vi "Launcher.vi"() -> ()   [LabVIEW 2012]
uses:
  State_Machine_Enum.ctl
  RefnameEnum.ctl
  Sally_Dashboard_2014/DBNameEnum.ctl
  Robot Global Data.vi
  <vilib>/addons/control/pid/pid.llb/PID (DBL).vi
  <vilib>/addons/control/pid/NI_PID_pid.lvlib
panel:
  out "Analog Signal":dbl(graph)
  in  "ControllerMultiplier":dbl=3000.0
  out "rpm":dbl
  out "motor output":dbl
  out "Time Chart":dbl(graph)
  out "Time Difference":dbl
  in  "Rate (unit/s)":dbl=10.0
  out "State":T1
  out "Value":dbl
  out "Stopped":bool
  out "MotorInput Chart":dbl(graph)=1.0
  out "RPM Chart":dbl(graph)=2105.9590349511814
  out "LauncherTargetRPM":dbl
  in  "PID gains":T2={"proportional gain (Kc)"=0.002, "integral time (Ti, min)"=0.005, "derivative time (Td, min)"=0.0} {"derivative time (Td, min)" step=0.0001 format="%.6f"; "integral time (Ti, min)" step=0.0001 format="%.6f"; "proportional gain (Kc)" step=0.0001 format="%.6f"}
  in  "output range":cluster{"output high":dbl, "output low":dbl}={"output high"=1.0, "output low"=0.0} {"output low" step=0.1 format="%.2f"; "output high" step=0.1 format="%.2f"}
  # "NOTE: UseEncoder\nmust be true in order\nto run PID"
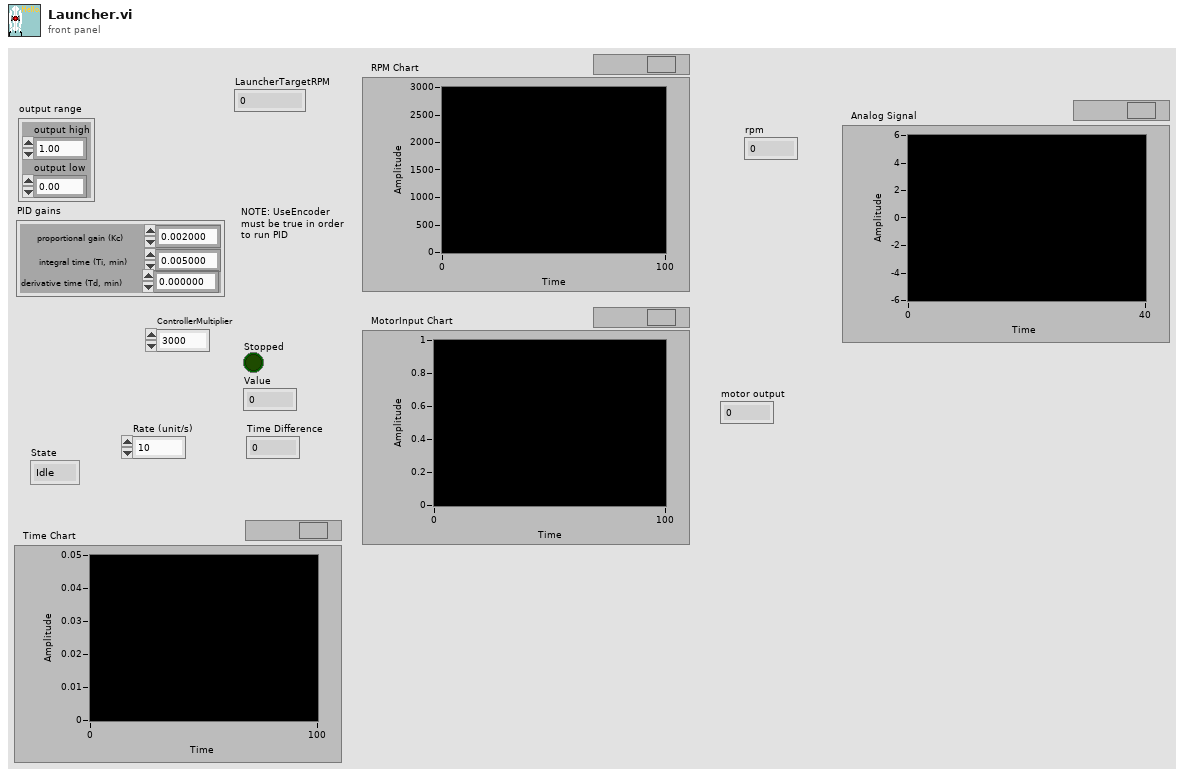
[diagram p1: front panel]
types:
  T1 = typedef "State_Machine_Enum.ctl" = enum16{"Idle", "Start", "Do", "Stop", "Init"}
  T2 = cluster{"proportional gain (Kc)":dbl, "integral time (Ti, min)":dbl, "derivative time (Td, min)":dbl}
  T3 = typedef "RefnameEnum.ctl" = enum16{"FireLauncher", "Climber", "Shield", "TankDrive", "DriveEncoderL", "DriveEncoderR", "LauncherMotorRPM", "LauncherEncoderAnalog", "LauncherEncoderRPM", "ShooterLS", "DriveAlignLSLeft", "DriveAlignLSRight", "ClimbingLS", "LauncherEncoderAngle", "LauncherMotorAngle", "Gamepad1", "Gamepad2", "Compressor", "ClimbWeightSol3", "ClimbWeightSol4"}
  T4 = typedef "DBNameEnum.ctl" = enum16{"AutoInstructions", "DriveLoopTime", "DriveAlignLSLeft", "DriveAlignLSRight", "Use2DriveAlign", "ClimbLS", "LauncherAngleMatches", "FrameworkVersion", "sLauncherAngle", "LauncherTargetAngle", "sLauncherRPM", "LauncherTargetRPM", "sDriveDistance", "LauncherMotorValue", "PullbackTol", "FireTol", "LauncherRPMTol", "LauncherAngleTol", "InitialWait", "WaitBetweenLaunch", "AnglePresets", "RPMPresets", "UseAngleEncoder", "UseLauncherEncoder", "UseLauncherPID", "QSWaitBeforeFire", "QSWaitBeforeRetract", "AngleForwardValue", "AngleBackwardValue", "UseClusterArray", "BackupAuto", "ReverseDriveIndicate", "HalfSpeedFactor"}
  T5 = typedef "LoopDisable.ctl" = cluster{"Climb.vi":bool, "LauncherAngle.vi":bool, "Launcher.vi":bool, "ArmControl.vi":bool, "WinchMotor.vi":bool, "ReadDriveEncoder.vi":bool}
  T6 = typedef "WPI_CounterDevRef.ctl" = cluster{"DevStatus":errorcluster, "CntIndex":T7}
  T7 = typedef "FPGA_CounterCtrSystemIndex.ctl" = enum8{"Ctr 0", "Ctr 1", "Ctr 2", "Ctr 3", "Ctr 4", "Ctr 5", "Ctr 6", "Ctr 7", "Invalid"}
  T8 = typedef "WPI_EncoderDevRef.ctl" = cluster{"DevStatus":errorcluster, "EncoderIndex":T9, "CounterIndex":T7, "DistancePerCount":dbl, "Decoding Type":T10}
  T9 = typedef "FPGA_EncoderIdx.ctl" = enum8{"Enc 0", "Enc 1", "Enc 2", "Enc 3", "Invalid"}
  T10 = typedef "WPI_EncoderType.ctl" = enum16{"1x", "2x", "4x"}
  T11 = typedef "WPI_AnalogChannelDevRef.ctl" = cluster{"DevStatus":errorcluster, "Analog Module":T12, "Analog Channel":T13}
  T12 = typedef "FPGA_TypedefAnalogModule.ctl" = enum16{"Analog Module 1", "Analog Module 2"}
  T13 = typedef "FPGA_AIChannel.ctl" = enum8{"AI 1", "AI 2", "AI 3", "AI 4", "AI 5", "AI 6", "AI 7", "AI 8", "Invalid"}
  T14 = typedef "WPI_MotorControlDeviceRef.ctl" = cluster{"DeviceStatus":errorcluster, "Type":enum16{"PWM", "CAN"}, "PWM":cluster{"Digital Module":T15, "PWM Channel":T16, "DeadBand":T17}, "CAN":cluster{"Device Number":u8, "Control Mode":T18, "Semaphore":T19, "Max Vout":dbl}, "Invert":bool, "TransformRef":T20, "InvTransformRef":T20}
  T15 = typedef "FPGA_TypedefDigitalModule.ctl" = enum16{"Digital Module 1", "Digital Module 2"}
  T16 = typedef "FPGA_DIOPWMChannel.ctl" = enum8{"PWM 1", "PWM 2", "PWM 3", "PWM 4", "PWM 5", "PWM 6", "PWM 7", "PWM 8", "PWM 9", "PWM 10", "Invalid"}
  T17 = typedef "WPI_PWMDeadband.ctl" = cluster{"Name":string, "maxPositivePwm":i32, "minPositivePwm":i32, "centerPwm":i32, "maxNegativePwm":i32, "minNegativePwm":i32, "angularRange":u16}
  T18 = typedef "WPI_CANJaguar_ControlMode.ctl" = enum8{"Percent VBus", "Current", "Speed", "Position", "Voltage"}
  T19 = typedef "Semaphore RefNum" = refnum<k1>
  T20 = typedef "WPI_PWMTransform_ConPane.ctl" = refnum<vi>
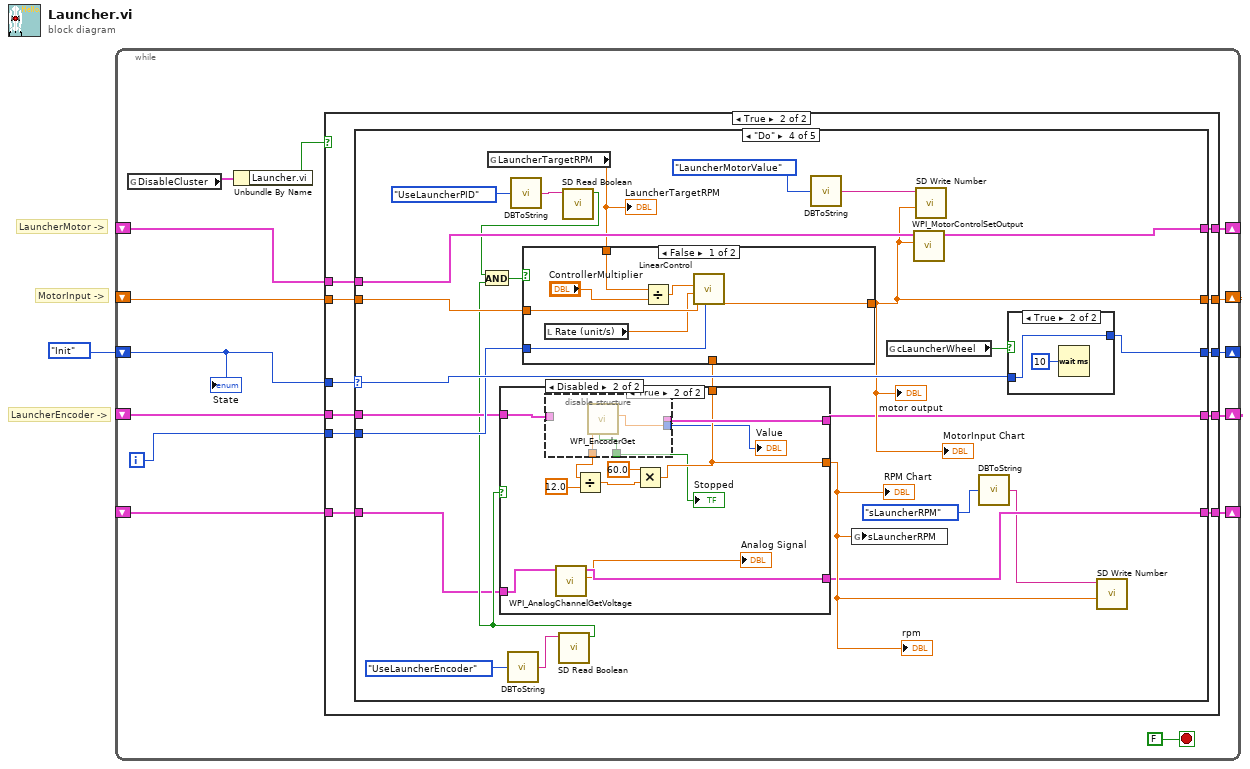
[diagram p0: block diagram]
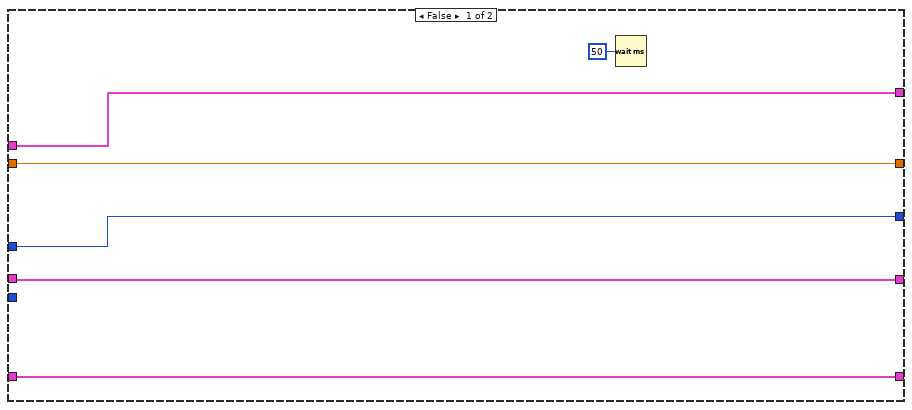
[diagram p2: hidden frame]
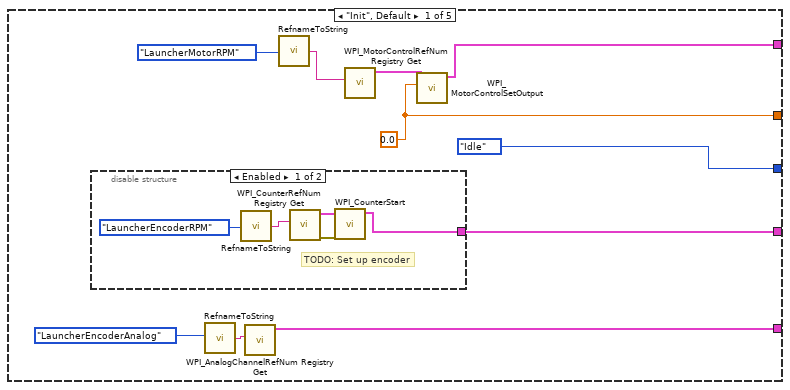
[diagram p3: hidden frame]
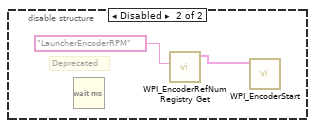
[diagram p4: hidden frame]
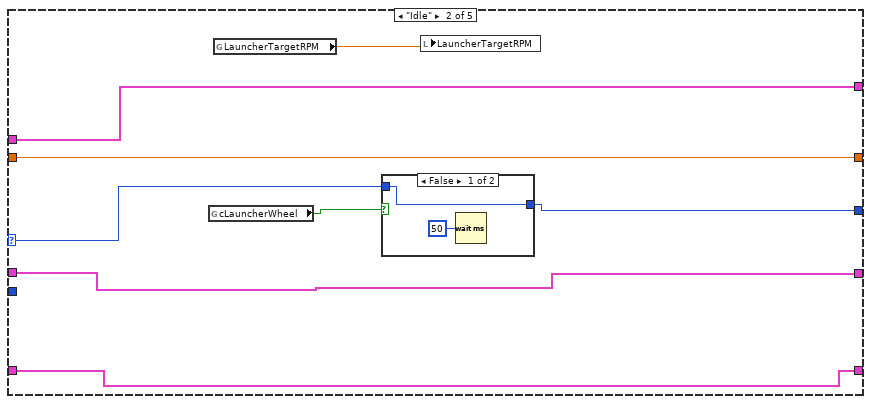
[diagram p5: hidden frame]
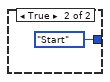
[diagram p6: hidden frame]
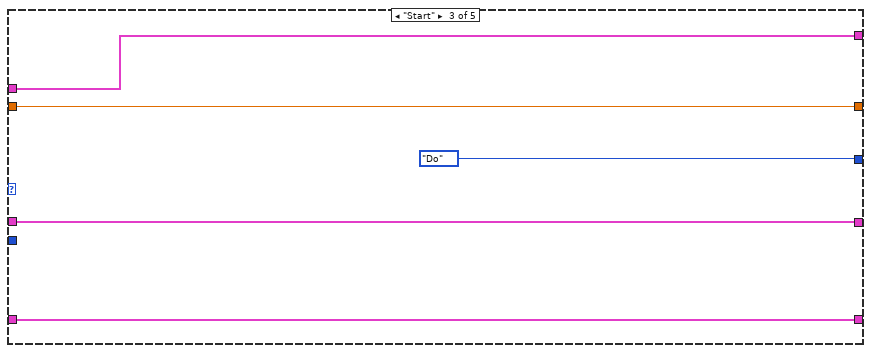
[diagram p7: hidden frame]
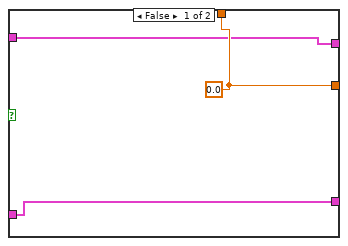
[diagram p8: hidden frame]
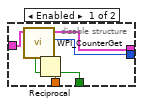
[diagram p9: hidden frame]
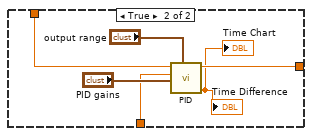
[diagram p10: hidden frame]
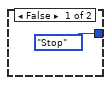
[diagram p11: hidden frame]
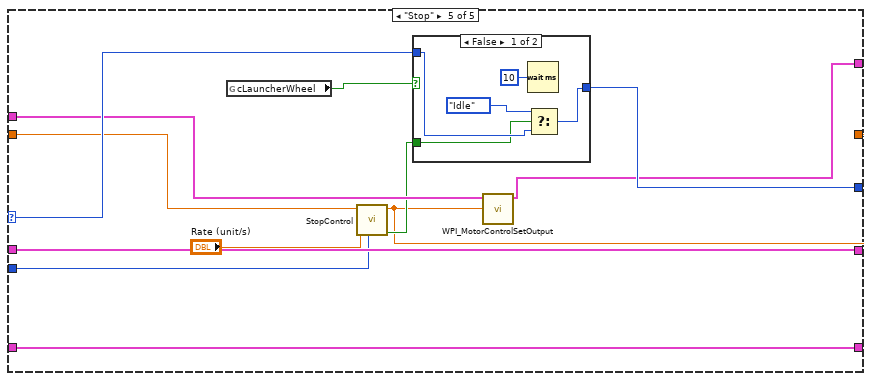
[diagram p12: hidden frame]
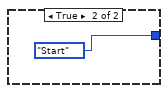
[diagram p13: hidden frame]
diagram:
  # "MotorInput ->"
  # "LauncherEncoder ->"
  # "LauncherMotor ->"
  n1 = while {
    shift-right: [w13] -> _
    shift-left: State_Machine_Enum."Init" ("State") -> [w14]
    shift-right: [w12] -> _
    shift-left: _ -> [w8]
    shift-right: [w11] -> _
    shift-left: _ -> [w9]
    shift-right: [w10] -> _
    shift-left: _ -> [w7]
    shift-right: [w3] -> _
    shift-left: _ -> [w2]
    i -> [w5]
    stop <- FALSE stop-if-true
    n2 = global read "Robot Global Data.vi" "DisableCluster"() -> (w6:T5)
    n3 = Unbundle By Name(w6) -> ("Launcher.vi"=w4:bool)
    n4 = case shown="True" w4 {
      tunnel: w14 -> [w19 w32]
      tunnel: [w19 w31] -> w13
      tunnel: [w18 w30] -> w12
      tunnel: [w21 w29] -> w11
      tunnel: [w20 w28] -> w10
      tunnel: w9 -> [w21 w27]
      tunnel: w8 -> [w18 w26]
      tunnel: w7 -> [w20 w25]
      tunnel: w5 -> [_ w24]
      tunnel: [w16 w23] -> w3
      tunnel: w2 -> [w16 w22]
      frame False {
        n5 = Wait (ms)(milliseconds to wait=u32 50) -> ()  [unwired: 1 out]
      }
      frame True {
        n6 = case shown="\"Do\"" w32 {
          selector: w32 -> [_ w56 _ w90 w143]
          tunnel: [State_Machine_Enum."Idle" ("State") w55 State_Machine_Enum."Do" ("State") w89 w142] -> w31
          tunnel: [w37 w50 w61 w81 w140] -> w30
          tunnel: [w41 w54 w65 w87 w139] -> w29
          tunnel: [w40 w53 w64 w83 w135] -> w28
          tunnel: w27 -> [_ w54 w65 w88 w138]
          tunnel: w26 -> [_ w50 w61 w82 w140]
          tunnel: w25 -> [_ w53 w64 w86 w137]
          tunnel: w24 -> [_ _ _ w85 w134]
          tunnel: [w38 w51 w62 w74 w132] -> w23
          tunnel: w22 -> [_ w51 w62 w75 w132]
          frame "Init", Default {
            w40 = 0.0 ("Output")
            n7 = disable-structure shown="Enabled" {
              disable-tunnel: [w45 _] -> w37
              frame Enabled {
                # "TODO: Set up encoder"
                n8 = call "RefnameToString.vi"("Enum"=RefnameEnum."LauncherEncoderRPM") -> ("Refname"=w43:string)
                n9 = call <vilib>:"WPI_CounterRefNum Registry Get.vi"("refnum name"=w43) -> ("error out"=w47:errorcluster, "CounterDevRef"=w46:T6)  [unwired: 9 in]
                n10 = call <vilib>:"WPI_CounterStart.vi"("error in (no error)"=w47, "CounterDevRef in"=w46) -> ("CounterDevRef out"=w45:T6)  [unwired: 8 in, 1 out]
              }
              frame Disabled {
                # "Deprecated"
                n11 = Wait (ms)() -> ()  [unwired: 1 in, 1 out]
                n12 = call <vilib>:"WPI_EncoderRefNum Registry Get.vi"("refnum name"="LauncherEncoderRPM") -> ("EncoderDevRef"=w48:T8)  [unwired: 9 in, 1 out]
                n13 = call <vilib>:"WPI_EncoderStart.vi"("EncoderDevRef"=w48) -> ()  [unwired: 9 in, 2 out]
              }
            }
            n14 = call "RefnameToString.vi"("Enum"=RefnameEnum."LauncherEncoderAnalog") -> ("Refname"=w33:string)
            n15 = call <vilib>:"WPI_AnalogChannelRefNum Registry Get.vi"("refnum name"=w33) -> ("AIDeviceRef"=w38:T11)  [unwired: 9 in, 1 out]
            n16 = call "RefnameToString.vi"("Enum"=RefnameEnum."LauncherMotorRPM") -> ("Refname"=w35:string)
            n17 = call <vilib>:"WPI_MotorControlRefNum Registry Get.vi"("refnum name"=w35) -> ("MotorControlDevRef"=w42:T14)  [unwired: 9 in, 1 out]
            n18 = call <vilib>:"WPI_MotorControlSetOutput.vi"("Output"=w40, "MotorControlDevRef"=w42) -> ("MotorControlDevRef"=w41:T14)  [unwired: 7 in, 2 out]
          }
          frame "Idle" {
            n19 = global read "Robot Global Data.vi" "cLauncherWheel"() -> (w57:bool)
            n20 = global read "Robot Global Data.vi" "LauncherTargetRPM"() -> (w52:dbl)
            n21 = case shown="False" w57 {
              tunnel: w56 -> [w58 _]
              tunnel: [w58 State_Machine_Enum."Start" ("State")] -> w55
              frame False {
                n22 = Wait (ms)(milliseconds to wait=u32 50) -> ()  [unwired: 1 out]
              }
              frame True {
              }
            }
            n23 = local write "LauncherTargetRPM"(w52) -> ()
          }
          frame "Start" {
          }
          frame "Do" {
            n24 = global read "Robot Global Data.vi" "LauncherTargetRPM"() -> (w84:dbl)
            "LauncherTargetRPM" <- w84
            n25 = call "DBToString.vi"("Enum"=DBNameEnum."UseLauncherEncoder") -> ("Refname"=w70:string)
            n26 = call "DBToString.vi"("Enum"=DBNameEnum."UseLauncherPID") -> ("Refname"=w72:string)
            n27 = call <vilib>:"SD Read Boolean.vi"("Name"=w70) -> ("Boolean"=w78:bool)  [unwired: 8 in, 2 out]
            n28 = case shown="True" w78 {
              tunnel: w82 -> [w93 w106]
              tunnel: [w93 w105] -> w81
              tunnel: [w94 w101] -> w80
              tunnel: [w94 w101] -> w76
              tunnel: w75 -> [w92 w97]
              tunnel: [w92 w96] -> w74
              frame False {
                w94 = 0.0
              }
              frame True {
                n29 = disable-structure shown="Disabled" {
                  disable-tunnel: w106 -> [w112 _]
                  disable-tunnel: [w111 _] -> w105
                  disable-tunnel: [w107 w113] -> w98
                  disable-tunnel: [w109 w115] -> w100
                  disable-tunnel: [w108 w114] -> w99
                  frame Enabled {
                    n30 = call <vilib>:"WPI_CounterGet.vi"("CounterDevRef in"=w112) -> ("Value"=w109:i32, "CounterDevRef out"=w111:T6, "Period (sec)"=w110:dbl, "Stopped"=w108:bool)  [unwired: 5 in, 2 out]
                    n31 = Reciprocal(x=w110) -> (1/x=w107:dbl)
                  }
                  frame Disabled {
                    n32 = call <vilib>:"WPI_EncoderGet.vi"() -> ("Distance"=w115:dbl, "Rate"=w113:dbl, "Stopped"=w114:bool)  [unwired: 6 in, 3 out]
                  }
                }
                "Stopped" <- w99
                "Value" <- w100
                n33 = call <vilib>:"WPI_AnalogChannelGetVoltage.vi"("AIDeviceRef"=w97) -> ("Voltage"=→"Analog Signal":dbl, "AIDeviceRef"=w96:T11)  [unwired: 8 in, 1 out]
                n34 = Divide(x=w98, y=12.0) -> (x/y=w103:dbl)
                n35 = Multiply(x=60.0, y=w103) -> (x*y=w101:dbl)
              }
            }
            "RPM Chart" <- w76
            "rpm" <- w76
            n36 = call <vilib>:"SD Read Boolean.vi"("Name"=w72) -> ("Boolean"=w77:bool)  [unwired: 8 in, 2 out]
            n37 = And(x=w77, y=w78) -> (x .and. y?=w79:bool)
            n38 = case shown="False" w79 {
              tunnel: w84 -> [w118 w128]
              tunnel: [w120 w127] -> w83
              tunnel: w86 -> [w119 _]
              tunnel: w85 -> [w117 _]
              tunnel: w80 -> [_ w124]
              frame False {
                n39 = local read "Rate (unit/s)"() -> (w116:dbl)
                n40 = Divide(x=w118, y="ControllerMultiplier") -> (x/y=w122:dbl)
                n41 = call "LinearControl.vi"("Loop Iteration"=w117, "Rate (unit/s)"=w116, "Setpoint"=w122, "Motor Value"=w119) -> ("New Motor Value"=w120:dbl)  [unwired: 6 in, 1 out]
              }
              frame True {
                n42 = call-poly <vilib>:"PID.vi"("output range"="output range", "PID gains"="PID gains", "process variable"=w124, "setpoint"=w128) -> ("dt out (s)"=→"Time Difference" →"Time Chart":dbl, "output"=w127:dbl)  [unwired: 6 in]
              }
            }
            "MotorInput Chart" <- w83
            "motor output" <- w83
            n43 = call "DBToString.vi"("Enum"=DBNameEnum."LauncherMotorValue") -> ("Refname"=w66:string)
            n44 = global write "Robot Global Data.vi" "sLauncherRPM"(w76) -> ()
            n45 = global read "Robot Global Data.vi" "cLauncherWheel"() -> (w91:bool)
            n46 = call <vilib>:"WPI_MotorControlSetOutput.vi"("Output"=w83, "MotorControlDevRef"=w88) -> ("MotorControlDevRef"=w87:T14)  [unwired: 7 in, 2 out]
            n47 = call <vilib>:"SD Write Number.vi"("Numeric"=w83, "Name"=w66) -> ()  [unwired: 8 in, 2 out]
            n48 = call "DBToString.vi"("Enum"=DBNameEnum."sLauncherRPM") -> ("Refname"=w69:string)
            n49 = case shown="True" w91 {
              tunnel: w90 -> [_ w130]
              tunnel: [State_Machine_Enum."Stop" ("State") w130] -> w89
              frame False {
              }
              frame True {
                n50 = Wait (ms)(milliseconds to wait=u32 10) -> ()  [unwired: 1 out]
              }
            }
            n51 = call <vilib>:"SD Write Number.vi"("Numeric"=w76, "Name"=w69) -> ()  [unwired: 8 in, 2 out]
          }
          frame "Stop" {
            n52 = global read "Robot Global Data.vi" "cLauncherWheel"() -> (w141:bool)
            n53 = call "StopControl.vi"("Loop Iteration"=w134, "Rate (unit/s)"="Rate (unit/s)", "Motor Value"=w137) -> ("Done Stopping"=w136:bool, "New Motor Value"=w135:dbl)  [unwired: 7 in]
            n54 = case shown="False" w141 {
              tunnel: w143 -> [w146 _]
              tunnel: [w145 State_Machine_Enum."Start" ("State")] -> w142
              tunnel: w136 -> [w144 _]
              frame False {
                n55 = Wait (ms)(milliseconds to wait=u32 10) -> ()  [unwired: 1 out]
                n56 = Select(t=State_Machine_Enum."Idle" ("State"), s=w144, f=w146) -> (s? t:f=w145:T1)
              }
              frame True {
              }
            }
            n57 = call <vilib>:"WPI_MotorControlSetOutput.vi"("Output"=w135, "MotorControlDevRef"=w138) -> ("MotorControlDevRef"=w139:T14)  [unwired: 7 in, 2 out]
          }
        }
      }
    }
    "State" <- w14
  }
